vi "Test Draw Snake.vi"(8 "error in (no error)":errorcluster, 11 "Test Case In":refnum<class "Snake Test.lvclass">) -> (0 "error out":errorcluster, 3 "Test Case Out":refnum<class "Snake Test.lvclass">)   [LabVIEW 2020, in "Snake Test.lvclass"]
uses:
  Snake Test.lvclass
  C:/Program Files (x86)/National Instruments/LabVIEW 2020/vi.lib/Astemes/LUnit/Test Case.lvclass
  source/Particle/Position.ctl
  source/Snake/Direction.ctl
  <vilib>/Astemes/LUnit/Test Case.lvclass/Test Case.ctl
  23f78a07-e948-4231-bc7c-64e7d42433eb.vi
  01074fa8-ee8a-411d-bc8b-fc92c4f90959.vi
  <vilib>/Astemes/LUnit/Set Assertion Type.vi
  <vilib>/Astemes/LUnit/Palette/Pass.vi
  <vilib>/Astemes/LUnit/Palette/Fail.vi
  <vilib>/Astemes/LUnit/Compare Variants.vi
  <vilib>/Astemes/LUnit/Describe Comparison.vi
  <vilib>/Astemes/LUnit/Add test result.vi
  <vilib>/Astemes/LUnit/Variant to string.vi
  <vilib>/Astemes/LUnit/LUnit Record Assertion Result.vi
  <vilib>/Astemes/LUnit/LUnit Aggregate Assertion Results.vi
  <vilib>/Astemes/LUnit/Method Result/LUnit Merge Status.vi
  <vilib>/Astemes/LUnit/LUnit Concatenate result strings.vi
  <vilib>/Utility/Data Type/Get Type Information.vi
  <vilib>/Utility/LVClass/Get LV Class Name.vi
  <vilib>/Comparison/Less/Less Functor/Less Functor.lvclass
  source/Snake/Snake.lvclass
  source/Particle.lvclass
  <vilib>/Astemes/LUnit/Test Case.lvclass
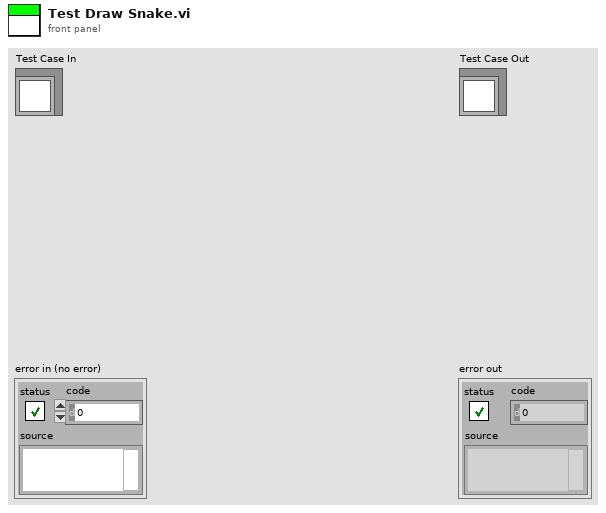
[diagram p1: front panel]
types:
  T1 = typedef "Snake.lvclass/Direction.ctl" = enum16{"X", "-X", "Y", "-Y"}
  T2 = typedef "Particle.lvclass/Position.ctl" = cluster{"X":i32, "Y":i32}
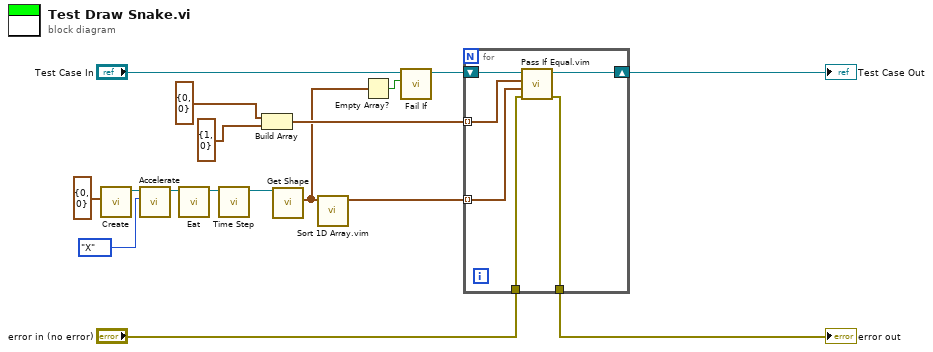
[diagram p0: block diagram]
diagram:
  n1 = call "Create.vi"("Position"=T2 {"X"=0, "Y"=0}) -> ("Snake out"=w17:refnum<class "Snake.lvclass">)  [unwired: 10 in]
  n2 = call "Accelerate.vi"("Direction"=Direction."X", "Snake in"=w17) -> ("Snake out"=w16:refnum<class "Snake.lvclass">)  [unwired: 9 in]
  n3 = call "Eat.vi"("Snake in"=w16) -> ("Snake out"=w15:refnum<class "Snake.lvclass">)  [unwired: 10 in]
  n4 = call "Time Step.vi"("Snake in"=w15) -> ("Snake out"=w12:refnum<class "Snake.lvclass">)  [unwired: 10 in]
  n5 = Build Array(cluster{"X":i32, "Y":i32} {"X"=0, "Y"=0} ("Position"), cluster{"X":i32, "Y":i32} {"X"=1, "Y"=0} ("Position")) -> (w8:cluster{"X":i32, "Y":i32}[])
  n6 = call-dynamic "Get Shape.vi"("Snake in"=w12) -> ("Coordinates"=w2:cluster{"X":i32, "Y":i32}[])  [unwired: 8 in, 2 out]
  n7 = call "Sort 1D Array.vim"("unsorted array"=w2) -> ("sorted array"=w9:cluster{"X":i32, "Y":i32}[])  [unwired: 10 in]
  n8 = Empty Array?(array=w2) -> (empty?=w1:bool)
  n9 = call <vilib>:"Fail If.vi"("Fail?"=w1, "LUnit Test Case In"="Test Case In") -> ("LUnit Test Case Out"=w3:refnum<class "Snake Test.lvclass">)  [unwired: 8 in, 1 out]
  n10 = for {
    tunnel: w9 -> [w18] mode=indexing
    tunnel: w8 -> [w19] mode=indexing
    tunnel: "error in (no error)" -> [w23]
    tunnel: [w21] -> w5
    shift-right: [w20] -> w4
    shift-left: w3 -> [w22]
    n11 = call "Pass If Equal.vim"("error in (no error)"=w23, "Actual"=w18, "Expected"=w19, "LUnit Test Case In"=w22) -> ("error out"=w21:errorcluster, "LUnit Test Case Out"=w20:refnum<class "Snake Test.lvclass">)  [unwired: 6 in]
  }
  "error out" <- w5
  "Test Case Out" <- w4
